vi "Is Named Bundler.vi"(10 "User VI Ref":refnum<vi>, 11 "Affected Items":T1) -> (0 "Terminal Ct":i32, 1 "First Term Selected":bool, 2 "Bundler Type":T2(ring), 3 "Named Cluster Un/bundle Selected":bool, 4 "EventBundler?":bool, 5 "Selected Term Ref":refnum<vi>, 6 "Data Type":variant)   [LabVIEW 2023]
doc: "Determine if selected BD object is a named bundler or unbundler with available elements to display (wired to a data source or sink)\n\nIf selected node is a cluster, then the output for the named bundler will be false, and the output for \"Is Cluster Node\" will be true. This ensures we have only one possible Affected Item type to work with.\n\nWe only consider element nodes on the (un)bundlers. The cluster input and output terminals are handled separately."
uses:
  top/BundleMagic.ctl
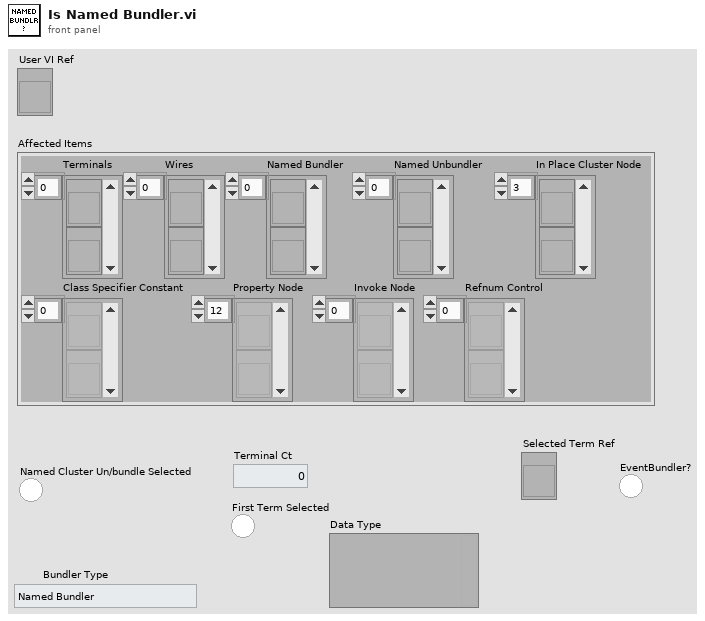
[diagram p1: front panel]
types:
  T1 = typedef "BundleMagic.ctl" = cluster{"Terminals":refnum<vi>[], "Wires":refnum<vi>[], "Named Bundler":refnum<vi>[], "Named Unbundler":refnum<vi>[], "In Place Cluster Node":refnum<vi>[], "Class Specifier Constant":refnum<vi>[], "Property Node":refnum<vi>[], "Invoke Node":refnum<vi>[], "Refnum Control":refnum<vi>[]}
  T2 = enum16{"Named Bundler", "Named Unbundler", "In Place", "None"}
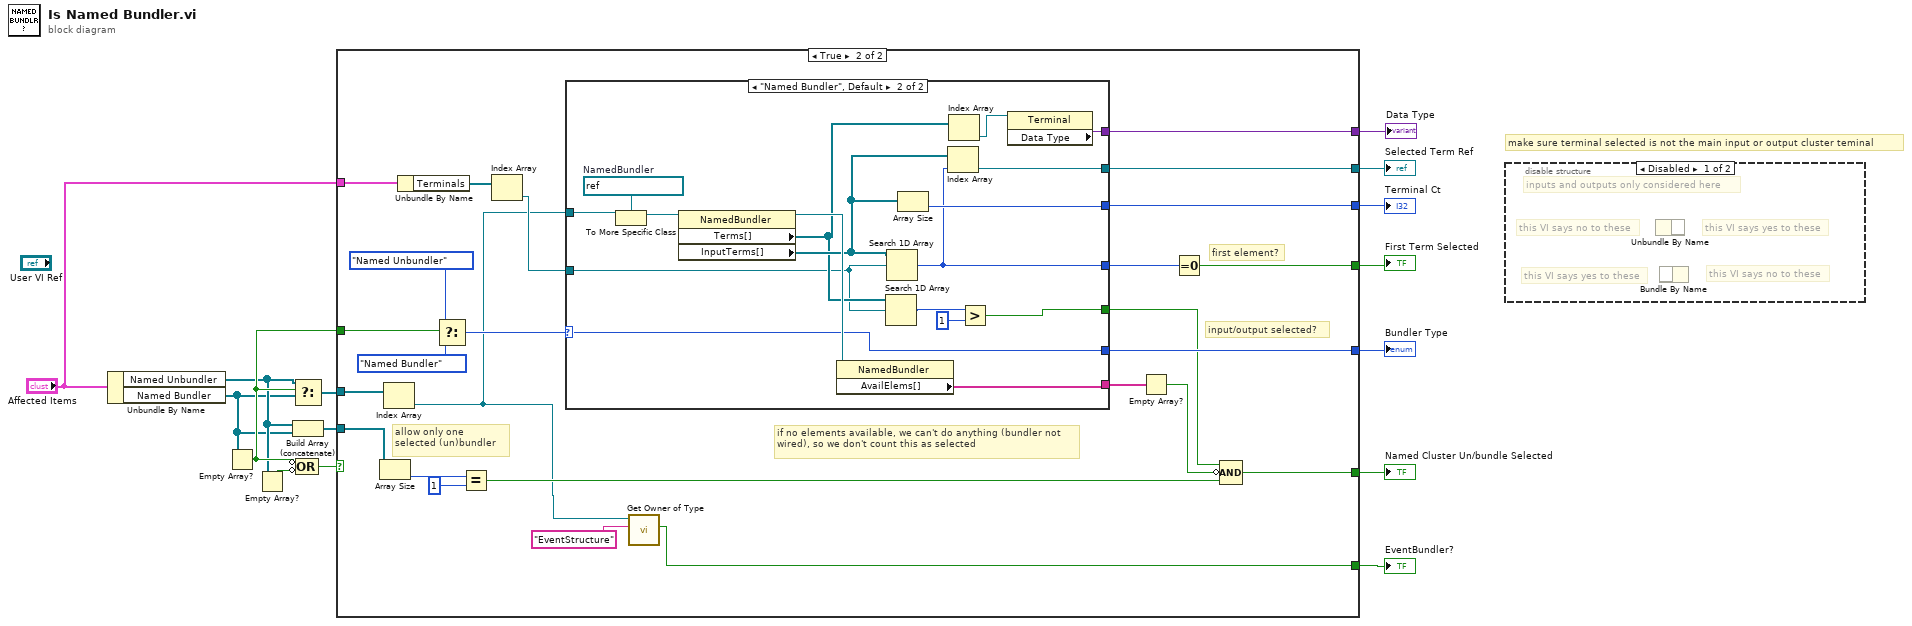
[diagram p0: block diagram]
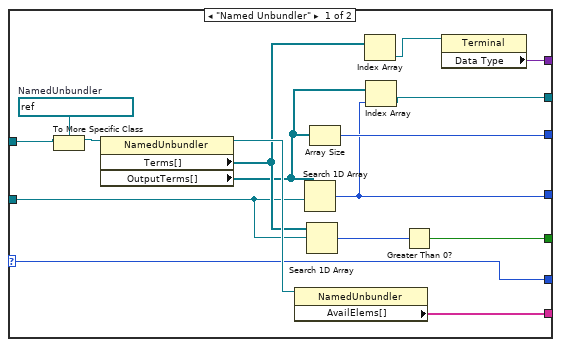
[diagram p3: hidden frame]
diagram:
  # "make sure terminal selected is not the main input or output cluster teminal"
  n1 = Unbundle By Name("Affected Items") -> ("Named Unbundler"=w4:refnum<vi>[], "Named Bundler"=w3:refnum<vi>[])
  n2 = Empty Array?(array=w3) -> (empty?=w5:bool)
  n3 = Empty Array?(array=w4) -> (empty?=w10:bool)
  n4 = Select(t=w4, s=w5, f=w3) -> (s? t:f=w8:refnum<vi>[])
  n5 = Build Array (concatenate)(w4, w3) -> (w2:refnum<vi>[])
  n6 = Compound Arithmetic op=OR(invert w5, invert w10) -> (w9:bool)
  n7 = case shown="True" w9 {
    tunnel: w8 -> [_ w23]
    tunnel: [_ w35] -> w15
    tunnel: [_ w34] -> w14
    tunnel: [_ w22] -> w13
    tunnel: [_ w33] -> w12
    tunnel: [_ w19] -> w11
    tunnel: "Affected Items" -> [_ w32]
    tunnel: [_ w25] -> w6
    tunnel: w5 -> [_ w29]
    tunnel: w2 -> [_ w24]
    tunnel: [_ w16] -> w1
    frame False {
    }
    frame True {
      # "input/output selected?"
      # "first element?"
      # "allow only one selected (un)bundler"
      # "if no elements available, we can't do anything (bundler not wired), so we don't count this as selected"
      n8 = Array Size(array=w24) -> (size(s)=w40:i32)
      n9 = Index Array(array=w23) -> (element=w17:refnum<vi>)  [unwired: 1 in]
      n10 = Unbundle By Name(w32) -> ("Terminals"=w31:refnum<vi>[])
      n11 = Select(t=T2."Named Unbundler" ("Bundler Type"), s=w29, f=T2."Named Bundler" ("Bundler Type")) -> (s? t:f=w26:T2)
      n12 = Equal?(x=w40, y=1) -> (x = y?=w36:bool)
      n13 = Index Array(array=w31) -> (element=w30:refnum<vi>)  [unwired: 1 in]
      n14 = case shown="\"Named Bundler\", Default" w26 {
        selector: w26 -> [w46 w66]
        tunnel: [w46 w66] -> w33
        tunnel: w17 -> [w56 w73]
        tunnel: w30 -> [w44 w60]
        tunnel: [w54 w71] -> w34
        tunnel: [w53 w70] -> w35
        tunnel: [w51 w68] -> w38
        tunnel: [w47 w64] -> w25
        tunnel: [w50 w62] -> w21
        tunnel: [w43 w57] -> w20
        frame "Named Unbundler" {
          w55 = refnum<vi> refnum  # NamedUnbundler
          n15 = To More Specific Class(target class=w55, reference=w56) -> (specific class reference=w49:refnum<vi>)  [unwired: 1 in, 1 out]
          n16 = property on="Property Node" class="NamedUnbundler"(reference=w49) -> (reference out=w52:refnum<vi>, "Terms[]"=w45:refnum<vi>[], "OutputTerms[]"=w41:refnum<vi>[])  [unwired: 1 in, 1 out]
          n17 = property on="Property Node" class="NamedUnbundler"(reference=w52) -> ("AvailElems[]"=w51:string[])  [unwired: 1 in, 2 out]
          n18 = Search 1D Array(1D array=w41, element=w44) -> (index of element=w50:i32)  [unwired: 1 in]
          n19 = Search 1D Array(1D array=w45, element=w44) -> (index of element=w42:i32)  [unwired: 1 in]
          n20 = Array Size(array=w41) -> (size(s)=w54:i32)
          n21 = Index Array(array=w45) -> (element=w48:refnum<vi>)  [unwired: 1 in]
          n22 = Index Array(array=w41, index=w50) -> (element=w53:refnum<vi>)
          n23 = Greater Than 0?(x=w42) -> (x > 0?=w43:bool)
          n24 = property on="Property Node" class="Terminal"(reference=w48) -> ("Data Type"=w47:variant)  [unwired: 1 in, 2 out]
        }
        frame "Named Bundler", Default {
          w72 = refnum<vi> refnum  # NamedBundler
          n25 = To More Specific Class(target class=w72, reference=w73) -> (specific class reference=w67:refnum<vi>)  [unwired: 1 in, 1 out]
          n26 = property on="Property Node" class="NamedBundler"(reference=w67) -> (reference out=w69:refnum<vi>, "Terms[]"=w61:refnum<vi>[], "InputTerms[]"=w63:refnum<vi>[])  [unwired: 1 in, 1 out]
          n27 = property on="Property Node" class="NamedBundler"(reference=w69) -> ("AvailElems[]"=w68:string[])  [unwired: 1 in, 2 out]
          n28 = Search 1D Array(1D array=w61, element=w60) -> (index of element=w59:i32)  [unwired: 1 in]
          n29 = Search 1D Array(1D array=w63, element=w60) -> (index of element=w62:i32)  [unwired: 1 in]
          n30 = Array Size(array=w63) -> (size(s)=w71:i32)
          n31 = Index Array(array=w63, index=w62) -> (element=w70:refnum<vi>)
          n32 = Index Array(array=w61) -> (element=w65:refnum<vi>)  [unwired: 1 in]
          n33 = Greater?(x=w59, y=1) -> (0:w57:bool)
          n34 = property on="Property Node" class="Terminal"(reference=w65) -> ("Data Type"=w64:variant)  [unwired: 1 in, 2 out]
        }
      }
      n35 = call "Get Owner of Type.vi"("Owner Class Name desired"="EventStructure", "reference"=w17) -> ("Owner of type found?"=w16:bool)  [unwired: 5 in, 4 out]
      n36 = Empty Array?(array=w38) -> (empty?=w37:bool)
      n37 = Equal To 0?(x=w21) -> (x = 0?=w22:bool)
      n38 = Compound Arithmetic op=AND(w20, invert w37, w36) -> (w19:bool)
    }
  }
  "Named Cluster Un/bundle Selected" <- w11
  "Bundler Type" <- w12
  "First Term Selected" <- w13
  "Terminal Ct" <- w14
  "Selected Term Ref" <- w15
  "Data Type" <- w6
  "EventBundler?" <- w1
  n39 = disable-structure shown="Disabled" {
    frame Disabled {
      # "inputs and outputs only considered here"
      # "this VI says no to these"
      # "this VI says yes to these"
      # "this VI says no to these"
      # "this VI says yes to these"
      n40 = Unbundle By Name() -> ()  [unwired: 1 in, 1 out]
      n41 = Bundle By Name() -> ()  [unwired: 2 in, 1 out]
    }
    frame Enabled {
    }
  }
